vi "Add New Message.vi"(8 "error in (no error)":errorcluster, 11 "Node Ptr":u64 format="%.0x") -> (0 "error out":errorcluster)   [LabVIEW 2019, in "Instrument Addon System Explorer.lvlib"]
uses:
  Instrument Addon System Explorer.lvlib
  <vilib>/NI VeriStand/Custom Device API/Custom Device Channel.ctl
  <vilib>/NI VeriStand/Custom Device API/Custom Device Channel Type.ctl
  Addon Shared/Constants.vi
  <vilib>/NI VeriStand/Custom Device API/Custom Device API.lvlib
  Addon Shared/Instrument Addon Shared.lvlib
panel:
  in  "Tag":string
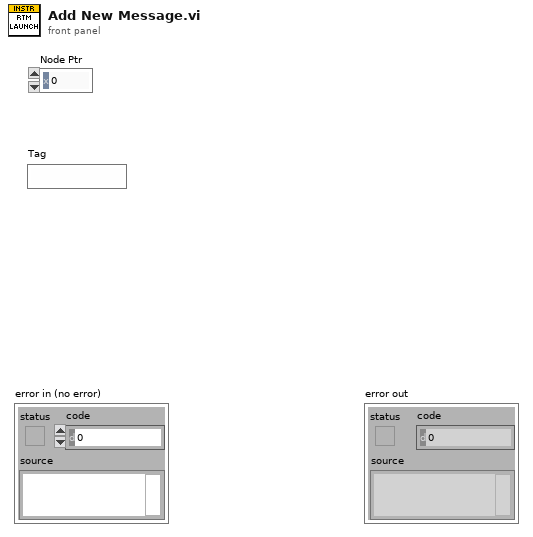
[diagram p1: front panel]
types:
  T1 = typedef "Custom Device API.lvlib/Custom Device Channel.ctl" = cluster{"Type":T2, "Units":string, "Default Value":dbl, "Faultable":bool, "Scalable":bool}
  T2 = typedef "Custom Device API.lvlib/Custom Device Channel Type.ctl" = enum16{"Input", "Output"}
  T3 = typedef "Custom Device API.lvlib/Custom Device Item Ref.ctl" = u64
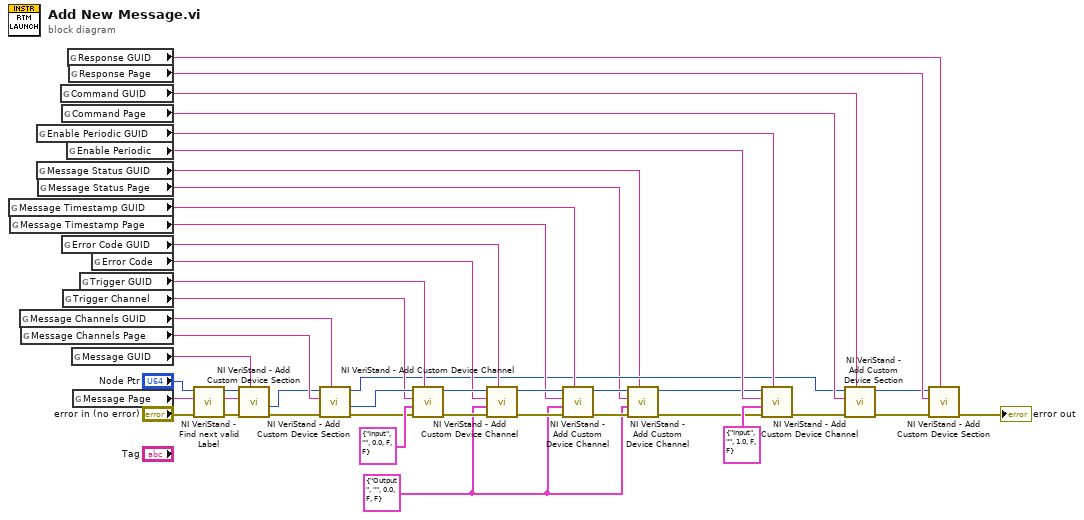
[diagram p0: block diagram]
diagram:
  w5 = T1 {"Type"=enum."Output", "Units"="", "Default Value"=0.0, "Faultable"=FALSE, "Scalable"=FALSE} ("Channel")
  n1 = global read "Constants.vi" "Message Timestamp GUID"() -> (w17:string)
  n2 = global read "Constants.vi" "Message Timestamp Page"() -> (w16:string)
  n3 = global read "Constants.vi" "Message Channels GUID"() -> (w34:string)
  n4 = global read "Constants.vi" "Message Channels Page"() -> (w35:string)
  n5 = global read "Constants.vi" "Enable Periodic GUID"() -> (w15:string)
  n6 = global read "Constants.vi" "Message Status GUID"() -> (w2:string)
  n7 = global read "Constants.vi" "Message Status Page"() -> (w1:string)
  n8 = global read "Constants.vi" "Command GUID"() -> (w23:string)
  n9 = global read "Constants.vi" "Command Page"() -> (w22:string)
  n10 = global read "Constants.vi" "Error Code GUID"() -> (w27:string)
  n11 = global read "Constants.vi" "Trigger Channel"() -> (w30:string)
  n12 = global read "Constants.vi" "Enable Periodic"() -> (w14:string)
  n13 = global read "Constants.vi" "Response GUID"() -> (w24:string)
  n14 = global read "Constants.vi" "Response Page"() -> (w25:string)
  n15 = global read "Constants.vi" "Message GUID"() -> (w36:string)
  n16 = global read "Constants.vi" "Message Page"() -> (w37:string)
  n17 = global read "Constants.vi" "Trigger GUID"() -> (w31:string)
  n18 = global read "Constants.vi" "Error Code"() -> (w26:string)
  n19 = call <vilib>:"NI VeriStand - Find next valid Label.vi"("error in (no error)"="error in (no error)", "Label"=w37, "Item Ref in"="Node Ptr") -> ("error out"=w41:errorcluster, "Label out"=w40:string, "Item Ref out"=w39:T3)  [unwired: 4 in, 2 out]
  n20 = call <vilib>:"NI VeriStand - Add Custom Device Section.vi"("GUID (Default Section)"=w36, "error in (no error)"=w41, "Section Name"=w40, "Parent Ref in"=w39) -> ("error out"=w10:errorcluster, "Section Ptr"=w9:T3)  [unwired: 4 in, 2 out]
  n21 = call <vilib>:"NI VeriStand - Add Custom Device Section.vi"("GUID (Default Section)"=w34, "error in (no error)"=w10, "Section Name"=w35, "Parent Ref in"=w9) -> ("error out"=w33:errorcluster, "Section Ptr"=w32:T3, "Parent Ref out"=w8:T3)  [unwired: 4 in, 1 out]
  n22 = call <vilib>:"NI VeriStand - Add Custom Device Channel.vi"("GUID (Default Channel)"=w31, "error in (no error)"=w33, "Channel"=T1 {"Type"=enum."Input", "Units"="", "Default Value"=0.0, "Faultable"=FALSE, "Scalable"=FALSE}, "Channel Name"=w30, "Parent Ref in"=w32) -> ("error out"=w29:errorcluster, "Parent Ref out"=w28:T3)  [unwired: 3 in, 2 out]
  n23 = call <vilib>:"NI VeriStand - Add Custom Device Channel.vi"("GUID (Default Channel)"=w27, "error in (no error)"=w29, "Channel"=w5, "Channel Name"=w26, "Parent Ref in"=w28) -> ("error out"=w19:errorcluster, "Parent Ref out"=w18:T3)  [unwired: 3 in, 2 out]
  n24 = call <vilib>:"NI VeriStand - Add Custom Device Channel.vi"("GUID (Default Channel)"=w17, "error in (no error)"=w19, "Channel"=w5, "Channel Name"=w16, "Parent Ref in"=w18) -> ("error out"=w7:errorcluster, "Parent Ref out"=w6:T3)  [unwired: 3 in, 2 out]
  n25 = call <vilib>:"NI VeriStand - Add Custom Device Channel.vi"("GUID (Default Channel)"=w2, "error in (no error)"=w7, "Channel"=w5, "Channel Name"=w1, "Parent Ref in"=w6) -> ("error out"=w4:errorcluster, "Parent Ref out"=w3:T3)  [unwired: 3 in, 2 out]
  n26 = call <vilib>:"NI VeriStand - Add Custom Device Channel.vi"("GUID (Default Channel)"=w15, "error in (no error)"=w4, "Channel"=T1 {"Type"=enum."Input", "Units"="", "Default Value"=1.0, "Faultable"=FALSE, "Scalable"=FALSE}, "Channel Name"=w14, "Parent Ref in"=w3) -> ("error out"=w12:errorcluster)  [unwired: 3 in, 3 out]
  n27 = call <vilib>:"NI VeriStand - Add Custom Device Section.vi"("GUID (Default Section)"=w23, "error in (no error)"=w12, "Section Name"=w22, "Parent Ref in"=w8) -> ("error out"=w21:errorcluster, "Parent Ref out"=w20:T3)  [unwired: 4 in, 2 out]
  n28 = call <vilib>:"NI VeriStand - Add Custom Device Section.vi"("GUID (Default Section)"=w24, "error in (no error)"=w21, "Section Name"=w25, "Parent Ref in"=w20) -> ("error out"=→"error out":errorcluster)  [unwired: 4 in, 3 out]
